vi "Stop Feeder.vi"(7 "Description":string, 8 "Command Info In":T1) -> (0 "Command Info Out":T1)   [LabVIEW 2019]
doc: "This template is useful for immediate subsystem actions that do not need deadband filtering\n\nBe sure to right-click and select New from Template and save with a new command name."
uses:
  <vilib>/Rock Robotics/WPI/Framework/Command Status Info.ctl
  <vilib>/Rock Robotics/WPI/Framework/Completion Status.ctl
  <vilib>/Rock Robotics/WPI/Framework/Completion Notifier.ctl
  Implementation/Feeder Setpoints.ctl
  Implementation/Feeder Operations.ctl
  Implementation/Feeder Published Globals.vi
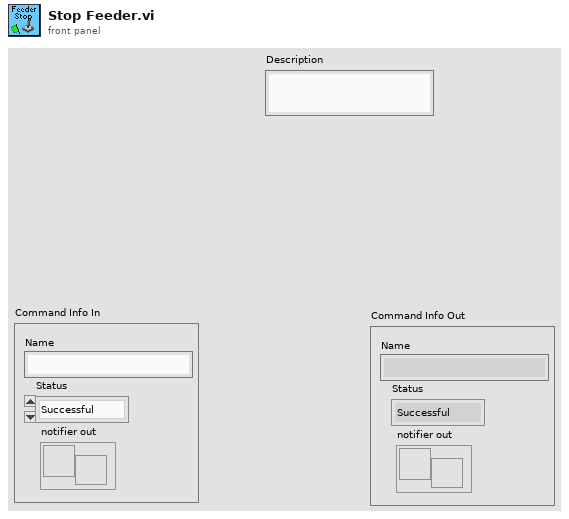
[diagram p1: front panel]
types:
  T1 = typedef "Command Status Info.ctl" = cluster{"Name":string, "Status":T2, "notifier out":T3}
  T2 = typedef "Completion Status.ctl" = enum16{"Successful", "Aborted", "Incomplete"}
  T3 = typedef "Completion Notifier.ctl" = refnum<notifier>
  T4 = typedef "Feeder Setpoints.ctl" = cluster{"Operation":T5, "Power":dbl, "Velocity":dbl, "Duration":dbl}
  T5 = typedef "Feeder Operations.ctl" = enum16{"Reserve", "Read Current", "Immediate", "Index Out Immediate", "Index In Immediate", "Start Feeder", "Index Out for Time", "Stop Feeder"}
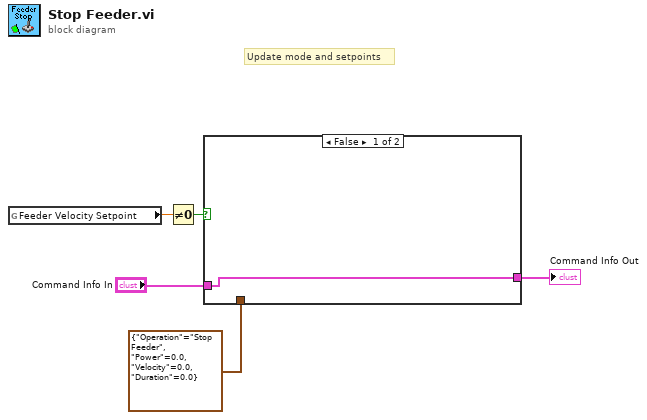
[diagram p0: block diagram]
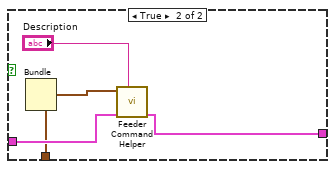
[diagram p2: hidden frame]
diagram:
  # "Update mode and setpoints"
  n1 = global read "Feeder Published Globals.vi" "Feeder Velocity Setpoint"() -> (w2:dbl)
  n2 = Not Equal To 0?(x=w2) -> (x != 0?=w3:bool)
  n3 = case shown="False" w3 {
    tunnel: "Command Info In" -> [w6 w11]
    tunnel: T4 {"Operation"=enum."Stop Feeder", "Power"=0.0, "Velocity"=0.0, "Duration"=0.0} ("SubSystem Data") -> [_ w9]
    tunnel: [w6 w7] -> w1
    frame False {
    }
    frame True {
      n4 = Bundle(cluster=w9) -> (w8:T4)  [unwired: 4 in]
      n5 = call "Feeder Command Helper.vi"("Description"="Description", "Command Info In"=w11, "SubSystem Data"=w8) -> ("Command Info Out"=w7:T1)  [unwired: 6 in, 2 out]
    }
  }
  "Command Info Out" <- w1
